vi "evo_irimager_set_focusmotor_pos.vi"(11 "Focus Pos %":sgl min=0 max=100) -> (3 "function return":i32)   [LabVIEW 2025, in "libirimager_direct_binding.lvlib"]
uses:
  GitHub/In-situ-monitoring-of-powder-bed-fusion-additive-manufacturing/system_development/Orichalcum/v0.2/Software_design/thermal-camera/VI/libirimager_direct_binding.lvlib
  GitHub/In-situ-monitoring-of-powder-bed-fusion-additive-manufacturing/system_development/Orichalcum/v0.2/Software_design/thermal-camera/VI/libirimager.dll
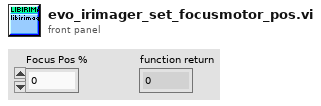
[diagram p1: front panel]
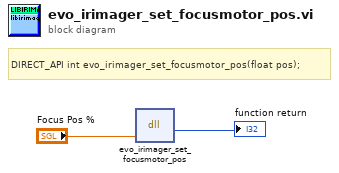
[diagram p0: block diagram]
diagram:
  # "DIRECT_API int evo_irimager_set_focusmotor_pos(float pos);"
  n1 = dll-call lib="C:/Users/mayhe/OneDrive/Documents/GitHub/In-situ-monitoring-of-powder-bed-fusion-additive-manufacturing/system_development/Orichalcum/v0.2/Software_design/thermal-camera/VI/libirimager.dll" fn="evo_irimager_set_focusmotor_pos"("pos"="Focus Pos %") -> ("Rückgabetyp"=→"function return":i32)  [unwired: 4 in, 2 out]
